vi "Add line to map.vi"(7 "Initial":sgl[][](array[numeric]), 8 "Read? (F)":bool, 9 "reset(f)":bool, 10 "Field index":i32, 11 "FDMR array":sgl[](array[numeric])) -> (1 "cols":i32, 2 "rows":i32, 3 "Map":sgl[][](array[numeric]))   [LabVIEW 2024]
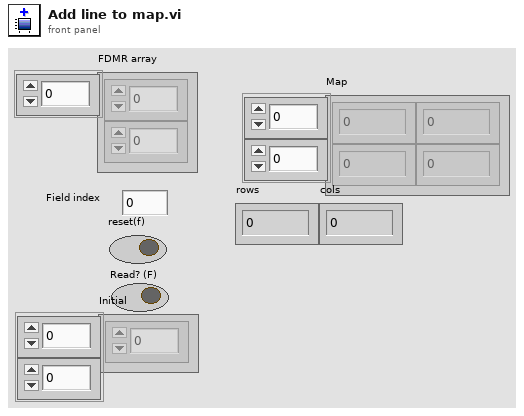
[diagram p1: front panel]
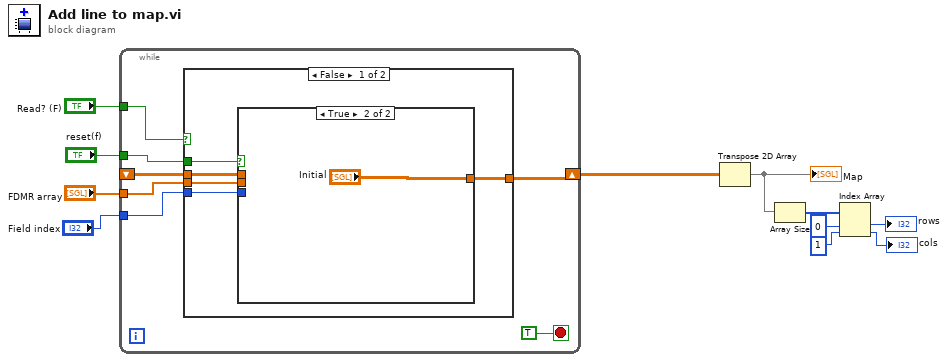
[diagram p0: block diagram]
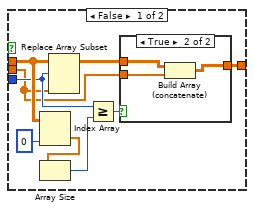
[diagram p2: hidden frame]
diagram:
  n1 = while {
    tunnel: "FDMR array" -> [w18]
    shift-right: [w14] -> w10
    shift-left: _ -> [w16]
    tunnel: "reset(f)" -> [w15]
    tunnel: "Read? (F)" -> [w13]
    tunnel: "Field index" -> [w12]
    stop <- TRUE stop-if-true
    n2 = case shown="False" w13 {
      tunnel: w18 -> [w23 _]
      tunnel: w16 -> [w22 w38]
      tunnel: w15 -> [w21 _]
      tunnel: [w20 w38] -> w14
      tunnel: w12 -> [w19 _]
      frame False {
        n3 = case shown="True" w21 {
          tunnel: w23 -> [w25 _]
          tunnel: [w24 "Initial"] -> w20
          tunnel: w22 -> [w32 _]
          tunnel: w19 -> [w28 _]
          frame False {
            n4 = Index Array(array=w32, index (col)=0 ("disabled index (col)")) -> (element=w30:sgl[])  [unwired: 1 in]
            n5 = Array Size(array=w30) -> (size(s)=w27:i32)
            n6 = Replace Array Subset(array=w32, new element=w25, index (row)=w28) -> (w26:sgl[][])  [unwired: 1 in]
            n7 = Greater Or Equal?(x=w28, y=w27) -> (x >= y?=w29:bool)
            n8 = case shown="True" w29 {
              tunnel: w26 -> [w33 w36]
              tunnel: w25 -> [_ w35]
              tunnel: [w33 w34] -> w24
              frame False {
              }
              frame True {
                n9 = Build Array (concatenate)(w36, w35) -> (w34:sgl[][])
              }
            }
          }
          frame True {
          }
        }
      }
      frame True {
      }
    }
  }
  n10 = Transpose 2D Array(2D array=w10) -> (transposed array=w8:sgl[][])
  "Map" <- w8
  n11 = Array Size(array=w8) -> (size(s)=w7:i32[])
  n12 = Index Array(array=w7, index #1=0 ("index"), index #2=1 ("index")) -> (element #1=→"rows":i32, element #2=→"cols":i32)
